vi "FindByTag.vi"(10 "Full Tag":string, 11 "Menu Item In":refnum<k24>) -> (2 "Found?":bool, 3 "Found Menu Item":refnum<k24>)   [LabVIEW 2016, in "MGI_TrayIcon.lvclass"]
doc: "Finds the references to the .NET menu item that corresponds to the full tag specififed.\n\nAuthored by Derek E. Trepanier\nsupport@mooregoodideas.com\nwww.mooregoodideas.com\n\nCopyright (c) 2012, Moore Good Ideas, Inc.\n\nAll rights reserved.\n\nRedistribution and use in source and binary forms, with or without modification, are permitted provided that the following conditions are met:\n\n * Redistributions of source code must retain the above copyright notice, this list of conditions and the following disclaimer.\n * Redistributions in binary form must reproduce the above copyright notice, this list of conditions and the following disclaimer in the documentation and/or other materials provided with the distribution.\n * Neither the name of Moore Good Ideas, Inc. nor the names of its contributors may be used to endorse or promote products derived from this software without specific prior written permission.\n\nTHIS SOFTWARE IS PROVIDED BY THE COPYRIGHT HOLDERS AND CONTRIBUTORS \"AS IS\" AND ANY EXPRESS OR IMPLIED WARRANTIES, INCLUDING, BUT NOT LIMITED TO, THE IMPLIED WARRANTIES OF MERCHANTABILITY AND FITNESS FOR A PARTICULAR PURPOSE ARE DISCLAIMED. IN NO EVENT SHALL THE COPYRIGHT OWNER OR CONTRIBUTORS BE LIABLE FOR ANY DIRECT, INDIRECT, INCIDENTAL, SPECIAL, EXEMPLARY, OR CONSEQUENTIAL DAMAGES (INCLUDING, BUT NOT LIMITED TO, PROCUREMENT OF SUBSTITUTE GOODS OR SERVICES; LOSS OF USE, DATA, OR PROFITS; OR BUSINESS INTERRUPTION) HOWEVER CAUSED AND ON ANY THEORY OF LIABILITY, WHETHER IN CONTRACT, STRICT LIABILITY, OR TORT (INCLUDING NEGLIGENCE OR OTHERWISE) ARISING IN ANY WAY OUT OF THE USE OF THIS SOFTWARE, EVEN IF ADVISED OF THE POSSIBILITY OF SUCH DAMAGE."
uses:
  <userlib>/_MGI/Menu Building/MenuTypes/TrayIcon/MGI_TrayIcon.lvclass
  System.Windows.Forms
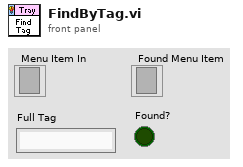
[diagram p1: front panel]
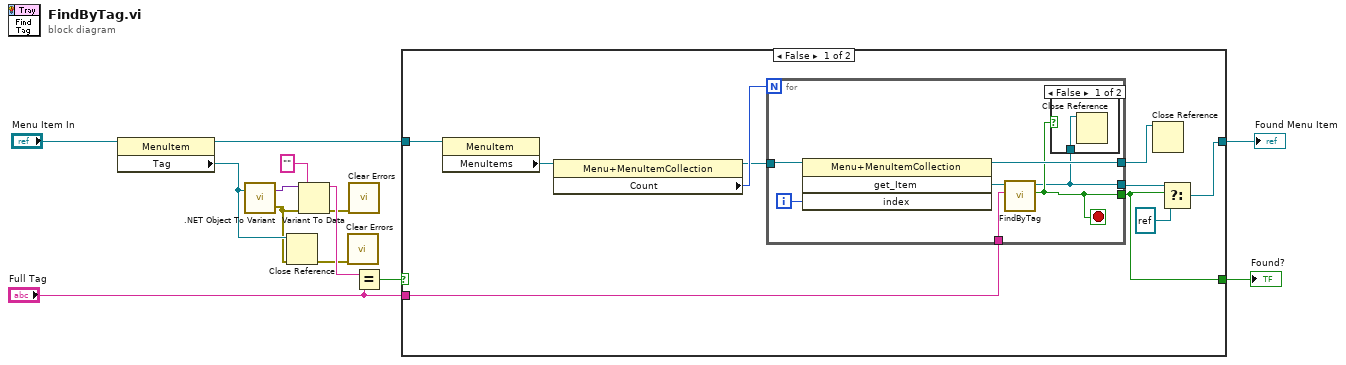
[diagram p0: block diagram]
diagram:
  n1 = property class="MenuItem"(reference="Menu Item In") -> (reference out=w9:refnum<k24>, "Tag"=w3:refnum<k24>)  [unwired: 1 in, 1 out]
  n2 = call <vilib>:".NET Object To Variant.vi"(".NET object"=w3) -> ("error out"=w2:errorcluster, "variant"=w12:variant)  [unwired: 1 in]
  n3 = Close Reference(reference=w3, error in (no error)=w2) -> (error out=w1:errorcluster)
  n4 = Variant To Data(error in=w2, type="", Variant=w12) -> (data=w10:string, error out=w4:errorcluster)
  n5 = call <vilib>:"Clear Errors.vi"("error in (no error)"=w1) -> ()  [unwired: 5 in, 2 out]
  n6 = call <vilib>:"Clear Errors.vi"("error in (no error)"=w4) -> ()  [unwired: 5 in, 2 out]
  n7 = Equal?(x=w10, y="Full Tag") -> (x = y?=w8:bool)
  n8 = case shown="False" w8 {
    selector: w8 -> [_ w32]
    tunnel: w9 -> [w23 w33]
    tunnel: [w16 w33] -> w7
    tunnel: [w15 w32] -> w6
    tunnel: "Full Tag" -> [w19 _]
    frame False {
      n9 = property class="MenuItem"(reference=w23) -> ("MenuItems"=w22:refnum<k24>)  [unwired: 1 in, 2 out]
      n10 = property class="Menu+MenuItemCollection"(reference=w22) -> (reference out=w20:refnum<k24>, "Count"=w21:i32)  [unwired: 1 in, 1 out]
      n11 = for {
        N: w21 -> [_]
        tunnel: w20 -> [w30]
        tunnel: w19 -> [w27]
        tunnel: [w24] -> w18
        tunnel: [w25] -> w15
        tunnel: [w26] -> w14
        i -> [w29]
        stop <- w25 stop-if-true
        n12 = invoke class="Menu+MenuItemCollection" method="get_Item"(reference=w30, "index"=w29) -> (reference out=w26:refnum<k24>, "get_Item"=w28:refnum<k24>)  [unwired: 2 in, 2 out]
        n13 = call <userlib>:"FindByTag.vi"("Full Tag"=w27, "Menu Item In"=w28) -> ("Found?"=w25:bool, "Found Menu Item"=w24:refnum<k24>)  [unwired: 8 in]
        n14 = case shown="False" w25 {
          tunnel: w24 -> [w31 _]
          frame False {
            n15 = Close Reference(reference=w31) -> ()  [unwired: 1 in, 1 out]
          }
          frame True {
          }
        }
      }
      n16 = Close Reference(reference=w14) -> ()  [unwired: 1 in, 1 out]
      n17 = Select(t=w18, s=w15, f=refnum<k24> refnum) -> (s? t:f=w16:refnum<k24>)
    }
    frame True {
    }
  }
  "Found Menu Item" <- w7
  "Found?" <- w6
